vi "UI  Update.vi"(8 "error in (no error)":errorcluster, 11 "Button_UI in":refnum<class "Button_UI.lvclass">) -> (0 "error out":errorcluster, 3 "Button_UI out":refnum<class "Button_UI.lvclass">)   [LabVIEW 2015, in "Button_UI.lvclass"]
uses:
  Button_UI.lvclass
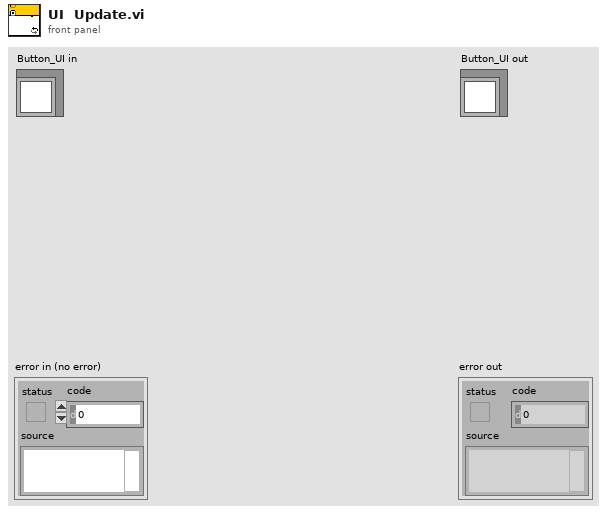
[diagram p1: front panel]
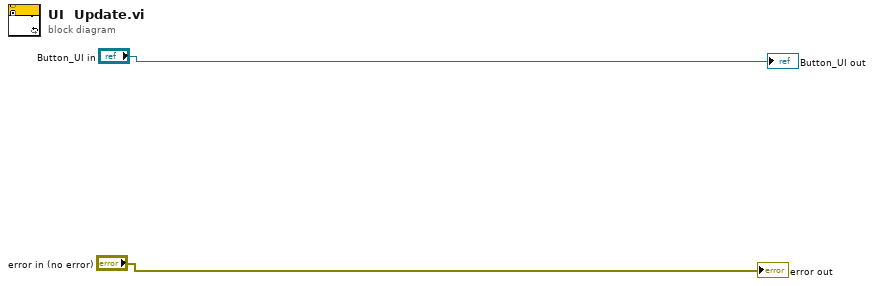
[diagram p0: block diagram]
diagram:
  "error out" <- "error in (no error)"
  "Button_UI out" <- "Button_UI in"
